vi "CRYAutoscale intervals.vi"(8 "No exact endpoints (F)":bool, 9 "Maximum ticks (12)":i32=12, 10 "Minimum value (0.0)":dbl format="%.2e", 11 "Maximum value":dbl format="%.2e") -> (0 "Number of ticks":i32, 1 "Tick interval":dbl format="%.2e", 2 "First tick":dbl format="%.2e", 3 "Tick values":dbl[](array[numeric]) format="%.2e", 4 "Scale max.":dbl format="%.2e", 6 "Scale min.":dbl format="%.2e")   [LabVIEW 2013]
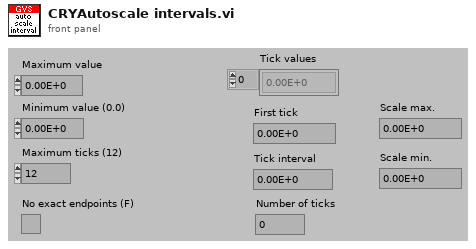
[diagram p1: front panel]
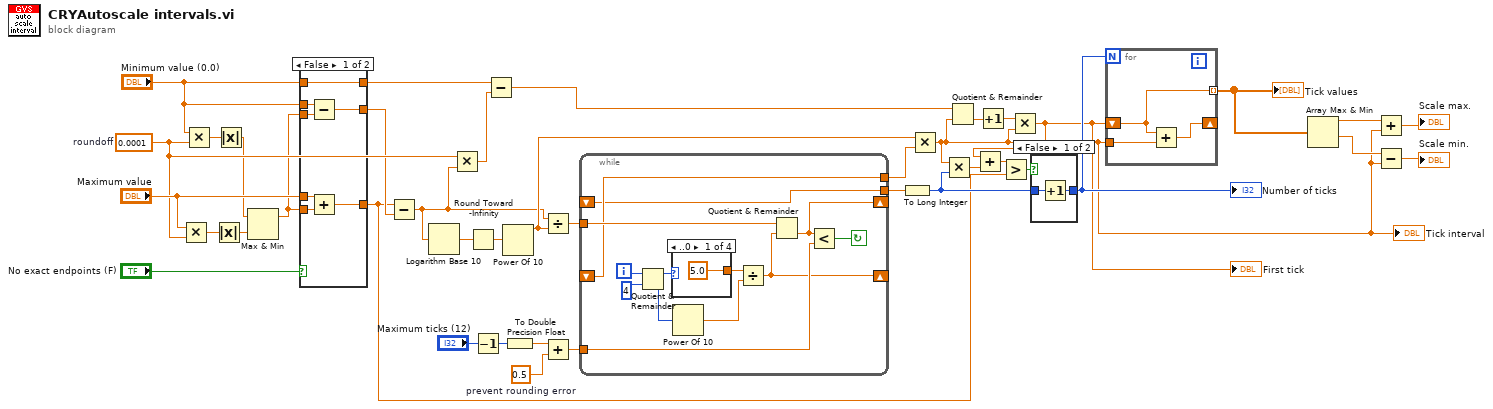
[diagram p0: block diagram]
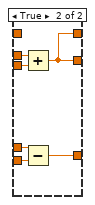
[diagram p2: hidden frame]
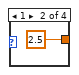
[diagram p4: hidden frame]
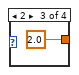
[diagram p5: hidden frame]
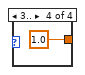
[diagram p6: hidden frame]
diagram:
  w30 = 0.5  # prevent rounding error
  w22 = 0.0001  # roundoff
  n1 = Multiply(x="Maximum value", y=w22) -> (x*y=w33:dbl)
  n2 = Multiply(x="Minimum value (0.0)", y=w22) -> (x*y=w35:dbl)
  n3 = Absolute Value(x=w33) -> (abs(x)=w11:dbl)
  n4 = Absolute Value(x=w35) -> (abs(x)=w10:dbl)
  n5 = Max & Min(x=w10, y=w11) -> (max(x,y)=w9:dbl)  [unwired: 1 out]
  n6 = case shown="False" "No exact endpoints (F)" {
    tunnel: "Maximum value" -> [w47 w53]
    tunnel: w9 -> [w46 w52]
    tunnel: w9 -> [w45 w51]
    tunnel: [w44 w48] -> w21
    tunnel: "Minimum value (0.0)" -> [w43 w50]
    tunnel: [w42 w49] -> w16
    tunnel: [w41 w48] -> w7
    tunnel: "Minimum value (0.0)" -> [w41 _]
    frame False {
      n7 = Subtract(x=w43, y=w46) -> (x-y=w44:dbl)
      n8 = Add(x=w47, y=w45) -> (x+y=w42:dbl)
    }
    frame True {
      n9 = Add(x=w50, y=w52) -> (x+y=w48:dbl)
      n10 = Subtract(x=w53, y=w51) -> (x-y=w49:dbl)
    }
  }
  n11 = Subtract(x=w16, y=w21) -> (x-y=w23:dbl)
  n12 = Logarithm Base 10(1:w23) -> (0:w40:dbl)
  n13 = Multiply(x=w22, y=w23) -> (x*y=w20:dbl)
  n14 = Round Toward -Infinity(1:w40) -> (0:w39:dbl)
  n15 = Decrement(x="Maximum ticks (12)") -> (x-1=w26:i32)
  n16 = Subtract(x=w7, y=w20) -> (x-y=w19:dbl)
  n17 = Power Of 10(x=w39) -> (10^x=w36:dbl)
  n18 = To Double Precision Float(number=w26) -> (double precision float=w31:dbl)
  n19 = Divide(x=w23, y=w36) -> (x/y=w28:dbl)
  n20 = Add(x=w31, y=w30) -> (x+y=w29:dbl)
  n21 = while {
    tunnel: w28 -> [w60]
    tunnel: w29 -> [w59]
    shift-right: [w57] -> _
    shift-left: _ -> [w56]
    tunnel: [w56] -> w37
    shift-right: [w55] -> _
    shift-left: _ -> [w54]
    tunnel: [w54] -> w32
    i -> [w66]
    stop <- w58 continue-if-true
    n22 = Quotient & Remainder(x=w66, y=4) -> (x-y*floor(x/y)=w64:i32, floor(x/y)=w63:i32)
    n23 = case shown="..0" w64 {
      tunnel: [5.0 2.5 2.0 1.0] -> w62
      frame ..0 {
      }
      frame 1 {
      }
      frame 2 {
      }
      frame 3.. {
      }
    }
    n24 = Power Of 10(x=w63) -> (10^x=w61:dbl)
    n25 = Divide(x=w62, y=w61) -> (x/y=w57:dbl)
    n26 = Quotient & Remainder(x=w60, y=w57) -> (floor(x/y)=w55:dbl)  [unwired: 1 out]
    n27 = Less?(x=w55, y=w59) -> (x < y?=w58:bool)
  }
  n28 = To Long Integer(number=w32) -> (32bit integer=w18:i32)
  n29 = Multiply(x=w36, y=w37) -> (x*y=w3:dbl)
  "Tick interval" <- w3
  n30 = Multiply(x=w3, y=w18) -> (x*y=w14:dbl)
  n31 = Quotient & Remainder(x=w19, y=w3) -> (floor(x/y)=w24:dbl)  [unwired: 1 out]
  n32 = Increment(x=w24) -> (x+1=w25:dbl)
  n33 = Multiply(x=w25, y=w3) -> (x*y=w15:dbl)
  "First tick" <- w15
  n34 = Add(x=w15, y=w14) -> (x+y=w13:dbl)
  n35 = Greater?(x=w13, y=w16) -> (0:w17:bool)
  n36 = case shown="False" w17 {
    tunnel: w18 -> [w72 w73]
    tunnel: [w71 w73] -> w27
    frame False {
      n37 = Increment(x=w72) -> (x+1=w71:i32)
    }
    frame True {
    }
  }
  "Number of ticks" <- w27
  n38 = for {
    N: w27 -> [_]
    shift-right: [w75] -> _
    shift-left: w15 -> [w74]
    tunnel: w3 -> [w76]
    tunnel: [w74] -> w6 mode=indexing
    n39 = Add(x=w74, y=w76) -> (x+y=w75:dbl)
  }
  "Tick values" <- w6
  n40 = Array Max & Min(array=w6) -> (max value=w5:dbl, min value=w4:dbl)  [unwired: 2 out]
  n41 = Add(x=w5, y=w3) -> (x+y=→"Scale max.":dbl)
  n42 = Subtract(x=w4, y=w3) -> (x-y=→"Scale min.":dbl)
